vi "doAction.vi"(8 "error in (no error)":errorcluster, 10 "ContextData":refnum<class "ContextData.lvclass">, 11 "Run in":refnum<class "Start Game.lvclass">) -> (0 "error out":errorcluster, 2 "ContextData Out":refnum<class "ContextData.lvclass">, 3 "Run out":refnum<class "Start Game.lvclass">)   [LabVIEW 2020, in "Start Game.lvclass"]
uses:
  Start Game.lvclass
  ContextData/ContextData.lvclass
  Player/Player.lvclass/Player.ctl
  Simon_Engine/Simon_Engine.lvclass
  Messages/simonMessages/simonMessages.lvclass
  uiControlsMgr/uiControlsMgr.lvclass
  Player/Player.lvclass
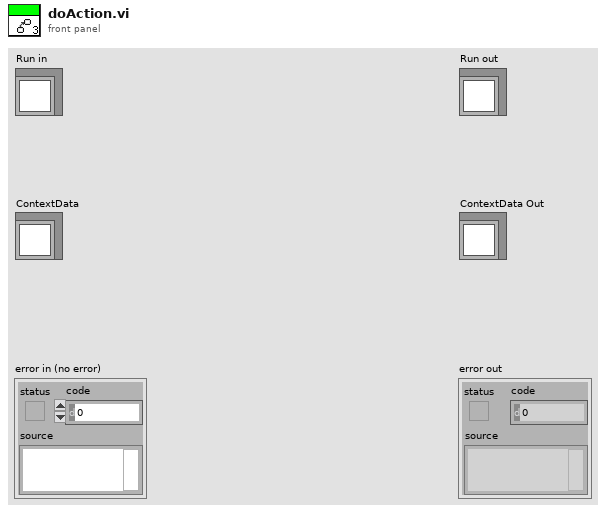
[diagram p1: front panel]
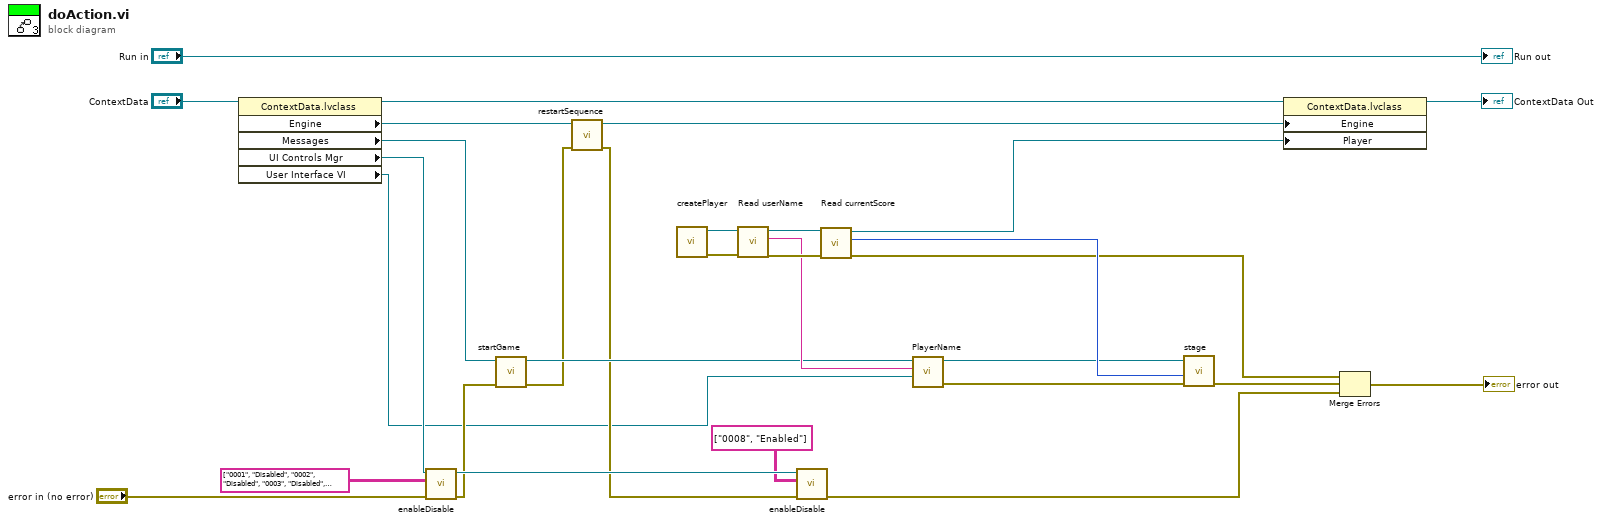
[diagram p0: block diagram]
diagram:
  n1 = property class="ContextData.lvclass"(reference="ContextData") -> (reference out=w20:refnum<class "ContextData.lvclass">, "Engine"=w12:refnum<class "Simon_Engine.lvclass">, "Messages"=w11:refnum<class "simonMessages.lvclass">, "UI Controls Mgr"=w6:refnum<class "uiControlsMgr.lvclass">, "User Interface VI"=w1:refnum<vi>)  [unwired: 1 in, 1 out]
  n2 = call "enableDisable.vi"("error in (no error)"="error in (no error)", "Controls - Status"=string[][] [["0001", "Disabled"], ["0002", "Disabled"], ["0003", "Disabled"], ["0004", "Disabled"], ["0005", "Disabled"], ["0006", "Disabled"], ["0007", "Disabled"]], "uiControlsMgr in"=w6) -> ("error out"=w5:errorcluster, "uiControlsMgr out"=w15:refnum<class "uiControlsMgr.lvclass">)  [unwired: 7 in]
  n3 = call "startGame.vi"("error in (no error)"=w5, "simonMessages in"=w11) -> ("error out"=w8:errorcluster, "simonMessages out"=w10:refnum<class "simonMessages.lvclass">)  [unwired: 8 in]
  n4 = call-dynamic "restartSequence.vi"("error in (no error)"=w8, "Simon_Engine in"=w12) -> ("error out"=w4:errorcluster, "Simon_Engine out"=w9:refnum<class "Simon_Engine.lvclass">)  [unwired: 8 in]
  n5 = call "createPlayer.vi"() -> ("error out"=w26:errorcluster, "Player out"=w29:refnum<class "Player.lvclass">)  [unwired: 10 in]
  n6 = call "Read userName.vi"("error in (no error)"=w26, "Player in"=w29) -> ("error out"=w27:errorcluster, "userName"=w22:string, "Player out"=w28:refnum<class "Player.lvclass">)  [unwired: 7 in]
  n7 = call "enableDisable.vi"("error in (no error)"=w4, "Controls - Status"=string[][] [["0008", "Enabled"]], "uiControlsMgr in"=w15) -> ("error out"=w3:errorcluster)  [unwired: 7 in, 1 out]
  n8 = call "Read currentScore.vi"("error in (no error)"=w27, "Player in"=w28) -> ("error out"=w18:errorcluster, "currentScore"=w25:u64, "Player out"=w13:refnum<class "Player.lvclass">)  [unwired: 7 in]
  n9 = call "PlayerName.vi"("VI Refnum"=w1, "PlayerName"=w22, "simonMessages in"=w10) -> ("error out"=w24:errorcluster, "simonMessages out"=w23:refnum<class "simonMessages.lvclass">)  [unwired: 7 in]
  n10 = call "stage.vi"("error in (no error)"=w24, "stage number"=w25, "simonMessages in"=w23) -> ("error out"=w17:errorcluster)  [unwired: 7 in, 1 out]
  n11 = property class="ContextData.lvclass"(reference=w20, "Engine"=w9, "Player"=w13) -> (reference out=→"ContextData Out":refnum<class "ContextData.lvclass">)  [unwired: 1 in, 1 out]
  n12 = Merge Errors(w18, w17, w3) -> (→"error out":errorcluster)
  "Run out" <- "Run in"
